vi "Take Single Reading.vi"(8 "error in (no error)":errorcluster, 11 "EPU452 in":refnum<class "EPU452.lvclass">) -> (0 "error out":errorcluster, 1 "Readings":dbl[](array[numeric]), 2 "Units":string[](array[string]), 3 "EPU452 out":refnum<class "EPU452.lvclass">, 5 "Response":string)   [LabVIEW 2018, in "EPU452.lvclass"]
uses:
  EPU452.lvclass
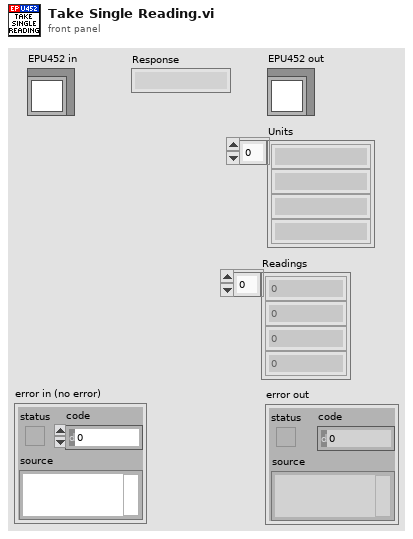
[diagram p1: front panel]
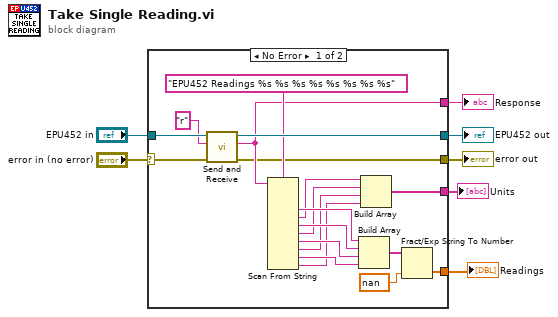
[diagram p0: block diagram]
diagram:
  n1 = case shown="No Error" "error in (no error)" {
    selector: "error in (no error)" -> [w21 w28]
    tunnel: [w13 w28] -> w6
    tunnel: [w17 w27] -> w4
    tunnel: "EPU452 in" -> [w22 w27]
    tunnel: [w15 _] -> w3
    tunnel: [w14 _] -> w2
    tunnel: [w8 _] -> w1
    frame No Error {
      n2 = call "Send and Receive.vi"("error in (no error)"=w21, "Command"="r", "EPU452 in"=w22) -> ("error out"=w13:errorcluster, "Response"=w14:string, "EPU452 out"=w17:refnum<class "EPU452.lvclass">)  [unwired: 6 in]
      n3 = Scan From String(format string="EPU452 Readings %s %s %s %s %s %s %s %s", input string=w14) -> (output 1=w26:string, output 2=w12:string, output 3=w25:string, output 4=w11:string, output 5=w24:string, output 6=w10:string, output 7=w23:string, output 8=w9:string)  [unwired: 10 in, 3 out]
      n4 = Build Array(w26, w25, w24, w23) -> (w19:string[])
      n5 = Build Array(w12, w11, w10, w9) -> (w8:string[])
      n6 = Fract/Exp String To Number(string=w19, default (0 dbl)=nan) -> (number=w15:dbl[])  [unwired: 2 in, 1 out]
    }
    frame Error {
    }
  }
  "error out" <- w6
  "EPU452 out" <- w4
  "Readings" <- w3
  "Response" <- w2
  "Units" <- w1
